vi "MediaCH.vi"(0 "input cluster":T1, 13 "Data":waveform(dbl)[](array[waveform])) -> (4 "Mitja CH1":dbl format="%0.2f", 6 "Mitja CH2":dbl format="%0.2f", 8 "Mitja CH3":dbl format="%0.2f", 10 "Mitja CH4":dbl format="%0.2f", 15 "Time Stamp":timestamp)   [LabVIEW 2014]
uses:
  <vilib>/Analysis/baseanly.llb/Mean (DBL).vi
  <vilib>/Waveform/WDTOps.llb/WDT Index Channel DBL.vi
  <vilib>/Analysis/NI_AALBase.lvlib
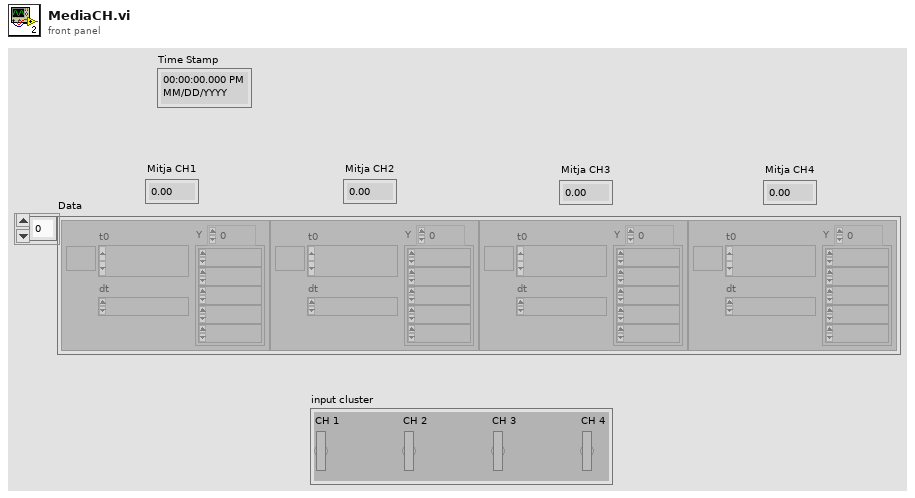
[diagram p1: front panel]
types:
  T1 = cluster{"CH 1":bool, "CH 2":bool, "CH 3":bool, "CH 4":bool}
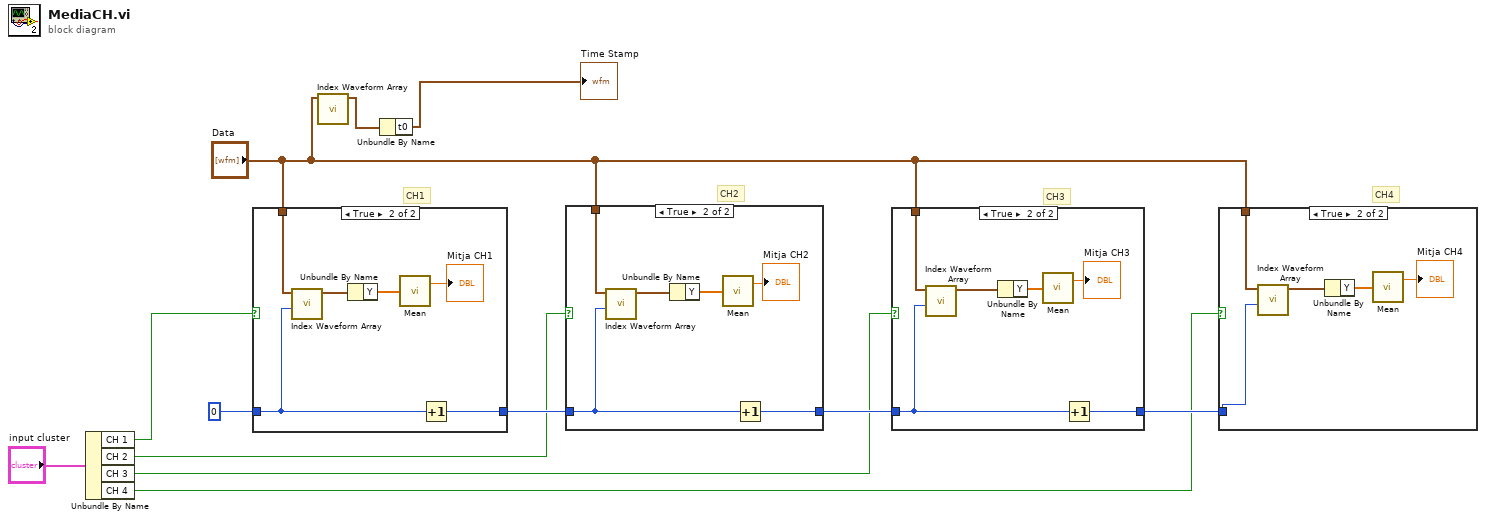
[diagram p0: block diagram]
diagram:
  # "CH4"
  # "CH3"
  # "CH2"
  # "CH1"
  n1 = Unbundle By Name("input cluster") -> ("CH 1"=w7:bool, "CH 2"=w6:bool, "CH 3"=w5:bool, "CH 4"=w4:bool)
  n2 = case shown="True" w7 {
    tunnel: 0 -> [w13 w18]
    tunnel: [w13 w17] -> w11
    tunnel: "Data" -> [_ w16]
    frame False {
    }
    frame True {
      n3 = call-poly <vilib>:"Index Waveform Array.vi"("index"=w18, "waveform array"=w16) -> ("waveform"=w15:waveform(dbl))  [unwired: 8 in, 1 out]
      n4 = Unbundle By Name(w15) -> ("Y"=w14:dbl[])
      n5 = call-poly <vilib>:"Mean.vi"("X"=w14) -> ("mean"=→"Mitja CH1":dbl)  [unwired: 1 out]
      n6 = Increment(x=w18) -> (x+1=w17:i32)
    }
  }
  n7 = call-poly <vilib>:"Index Waveform Array.vi"("waveform array"="Data") -> ("waveform"=w3:waveform(dbl))  [unwired: 9 in, 1 out]
  n8 = Unbundle By Name(w3) -> ("t0"=→"Time Stamp":timestamp)
  n9 = case shown="True" w6 {
    tunnel: w11 -> [w20 w26]
    tunnel: [w20 w25] -> w10
    tunnel: "Data" -> [_ w24]
    frame False {
    }
    frame True {
      n10 = call-poly <vilib>:"Index Waveform Array.vi"("index"=w26, "waveform array"=w24) -> ("waveform"=w22:waveform(dbl))  [unwired: 8 in, 1 out]
      n11 = Unbundle By Name(w22) -> ("Y"=w21:dbl[])
      n12 = call-poly <vilib>:"Mean.vi"("X"=w21) -> ("mean"=→"Mitja CH2":dbl)  [unwired: 1 out]
      n13 = Increment(x=w26) -> (x+1=w25:i32)
    }
  }
  n14 = case shown="True" w5 {
    tunnel: w10 -> [w27 w33]
    tunnel: [w27 w32] -> w9
    tunnel: "Data" -> [_ w31]
    frame False {
    }
    frame True {
      n15 = call-poly <vilib>:"Index Waveform Array.vi"("index"=w33, "waveform array"=w31) -> ("waveform"=w29:waveform(dbl))  [unwired: 8 in, 1 out]
      n16 = Unbundle By Name(w29) -> ("Y"=w28:dbl[])
      n17 = call-poly <vilib>:"Mean.vi"("X"=w28) -> ("mean"=→"Mitja CH3":dbl)  [unwired: 1 out]
      n18 = Increment(x=w33) -> (x+1=w32:i32)
    }
  }
  n19 = case shown="True" w4 {
    tunnel: w9 -> [_ w38]
    tunnel: "Data" -> [_ w37]
    frame False {
    }
    frame True {
      n20 = call-poly <vilib>:"Index Waveform Array.vi"("index"=w38, "waveform array"=w37) -> ("waveform"=w35:waveform(dbl))  [unwired: 8 in, 1 out]
      n21 = Unbundle By Name(w35) -> ("Y"=w34:dbl[])
      n22 = call-poly <vilib>:"Mean.vi"("X"=w34) -> ("mean"=→"Mitja CH4":dbl)  [unwired: 1 out]
    }
  }
